vi "tsc--Hex to Color.vi"(2 "Hex String":u32 format="%06x") -> (5 "Color":u32(colorbox)=14869218)   [LabVIEW 2021, in "Material SubVIs.lvlib"]
doc: "convert a hex representation of a color to RGB color box\n\n<b>Code Developed By:</b> +\nTechnology Service Corporation +\nwww.tsc.com/atcs +\n\nDeveloper: +\nDaniel Coons"
uses:
  Material SubVIs.lvlib
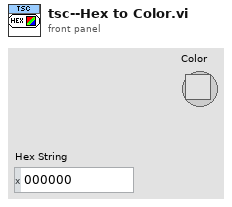
[diagram p1: front panel]
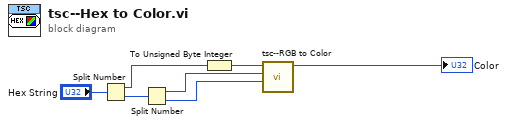
[diagram p0: block diagram]
diagram:
  n1 = Split Number(x="Hex String") -> (hi(x)=w4:u16, lo(x)=w5:u16)
  n2 = Split Number(x=w5) -> (hi(x)=w3:u8, lo(x)=w2:u8)
  n3 = To Unsigned Byte Integer(number=w4) -> (unsigned 8bit integer=w1:u8)
  n4 = call "tsc--RGB to Color.vi"("B"=w2, "G"=w3, "R"=w1) -> ("Color"=→"Color":u32)  [unwired: 8 in]
